vi "Stop.vi"(8 "error in (no error)":errorcluster, 11 "AudioGeneration in":refnum<class "AudioGeneration.lvclass">) -> (0 "error out":errorcluster, 3 "AudioGeneration out":refnum<class "AudioGeneration.lvclass">)   [LabVIEW 2021, in "AudioGeneration.lvclass"]
uses:
  AudioGeneration.lvclass
  AudioGeneration.lvclass/AudioGeneration.ctl
  <vilib>/NI/STM/NI STM.lvlib
  <vilib>/NI/STM/TCP/Write Message (TCP).vi
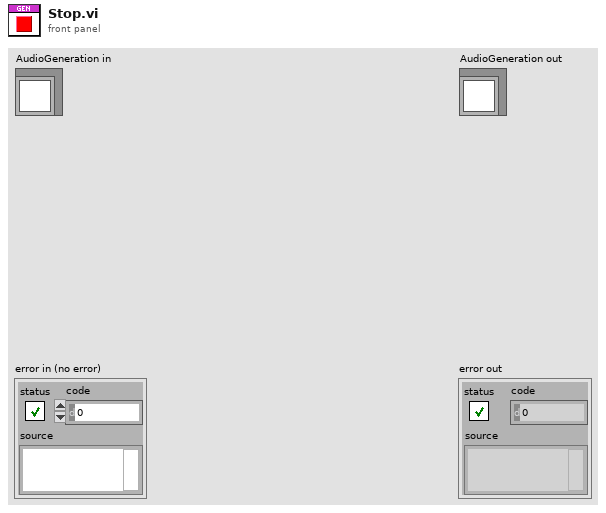
[diagram p1: front panel]
types:
  T1 = typedef "AudioGenTypeDefs.lvlib/generation type.ctl" = enum16{"analog", "digital"}
  T2 = typedef "NI STM.lvlib/TCP Connection Info.ctl" = cluster{"connection ID":refnum<k5>, "meta data":T3[]}
  T3 = typedef "NI STM.lvlib/MetaDataElement.ctl" = string
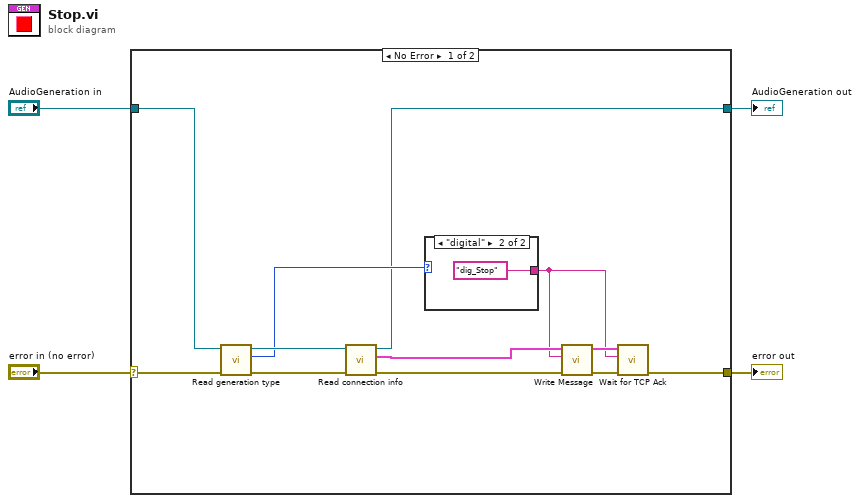
[diagram p0: block diagram]
diagram:
  n1 = case shown="No Error" "error in (no error)" {
    selector: "error in (no error)" -> [w8 w19]
    tunnel: [w5 w19] -> w3
    tunnel: [w6 w18] -> w1
    tunnel: "AudioGeneration in" -> [w7 w18]
    frame No Error {
      n2 = call-dynamic "Read generation type.vi"("error in (no error)"=w8, "AudioGeneration in"=w7) -> ("error out"=w16:errorcluster, "generation type"=w14:T1, "AudioGeneration out"=w15:refnum<class "AudioGeneration.lvclass">)  [unwired: 7 in]
      n3 = call-dynamic "Read connection info.vi"("error in (no error)"=w16, "AudioGeneration in"=w15) -> ("error out"=w13:errorcluster, "connection info"=w12:T2, "AudioGeneration out"=w6:refnum<class "AudioGeneration.lvclass">)  [unwired: 7 in]
      n4 = case shown="\"digital\"" w14 {
        tunnel: [_ "dig_Stop"] -> w9
        frame "analog", Default {
        }
        frame "digital" {
        }
      }
      n5 = call-poly <vilib>:"Write Message.vi"("error in"=w13, "name"=w9, "connection info in"=w12) -> ("error out"=w11:errorcluster, "connection info out"=w10:T2)  [unwired: 7 in]
      n6 = call "Wait for TCP Ack.vi"("error in (no error)"=w11, "cmd name"=w9, "connection info in"=w10) -> ("error out"=w5:errorcluster)  [unwired: 6 in, 2 out]
    }
    frame Error {
    }
  }
  "error out" <- w3
  "AudioGeneration out" <- w1
